vi "Play_Sound.vi"(1 "error in (no error)":errorcluster, 2 "Sound Type":i32) -> (0 "error out":errorcluster)   [LabVIEW 2015]
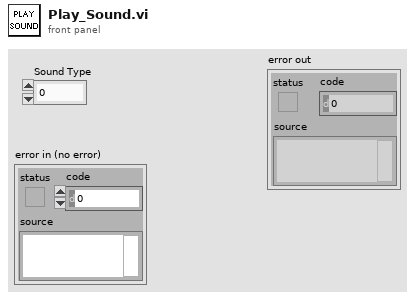
[diagram p1: front panel]
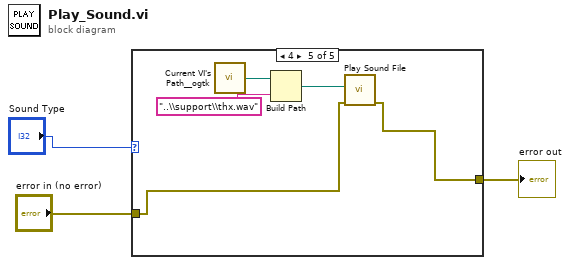
[diagram p0: block diagram]
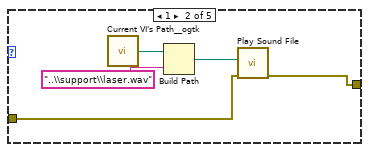
[diagram p3: hidden frame]
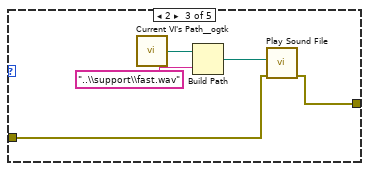
[diagram p4: hidden frame]
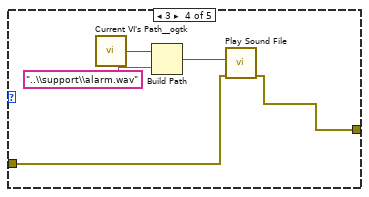
[diagram p5: hidden frame]
diagram:
  n1 = case shown="4" "Sound Type" {
    tunnel: "error in (no error)" -> [w4 w6 w11 w16 w21]
    tunnel: [w4 w5 w10 w15 w20] -> w1
    frame 0, Default {
    }
    frame 1 {
      n2 = call <userlib>:"Current VI's Path__ogtk.vi"() -> ("Current VI's Path (+ Relative)"=w9:path)  [unwired: 1 in]
      n3 = Build Path(base path=w9, name or relative path="..\\support\\laser.wav") -> (appended path=w7:path)
      n4 = call <vilib>:"Play Sound File.vi"("error in (no error)"=w6, "path"=w7) -> ("error out"=w5:errorcluster)  [unwired: 8 in, 1 out]
    }
    frame 2 {
      n5 = call <userlib>:"Current VI's Path__ogtk.vi"() -> ("Current VI's Path (+ Relative)"=w12:path)  [unwired: 1 in]
      n6 = Build Path(base path=w12, name or relative path="..\\support\\fast.wav") -> (appended path=w14:path)
      n7 = call <vilib>:"Play Sound File.vi"("error in (no error)"=w11, "path"=w14) -> ("error out"=w10:errorcluster)  [unwired: 8 in, 1 out]
    }
    frame 3 {
      n8 = call <userlib>:"Current VI's Path__ogtk.vi"() -> ("Current VI's Path (+ Relative)"=w17:path)  [unwired: 1 in]
      n9 = Build Path(base path=w17, name or relative path="..\\support\\alarm.wav") -> (appended path=w19:path)
      n10 = call <vilib>:"Play Sound File.vi"("error in (no error)"=w16, "path"=w19) -> ("error out"=w15:errorcluster)  [unwired: 8 in, 1 out]
    }
    frame 4 {
      n11 = call <userlib>:"Current VI's Path__ogtk.vi"() -> ("Current VI's Path (+ Relative)"=w22:path)  [unwired: 1 in]
      n12 = Build Path(base path=w22, name or relative path="..\\support\\thx.wav") -> (appended path=w24:path)
      n13 = call <vilib>:"Play Sound File.vi"("error in (no error)"=w21, "path"=w24) -> ("error out"=w20:errorcluster)  [unwired: 8 in, 1 out]
    }
  }
  "error out" <- w1
